vi "禹山叶绿素a校准.vi"() -> ()   [LabVIEW 2016, in "斯坦道多参数.lvlib"]
uses:
  <vilib>/Utility/miscctls.llb/LVPointTypeDef.ctl
  <vilib>/Analysis/NI_AALBase.lvlib
  <vilib>/Analysis/NI_AALPro.lvlib
  <vilib>/Utility/config.llb/NI_LVConfig.lvlib
panel:
  out "第二点校准值":dbl
  out "第一点校准值":dbl
  out "最小值":sgl format="%.2g"
  out "最大值":sgl format="%.2g"
  in  "校准停止":bool
  in  "校准模式":enum16{"两点校准", "单点校准"}(ring)
  in  "标液2":dbl
  in  "标液1":dbl
  out "波形图表":sgl(graph) caption="历史曲线"
  out "温度测量值":dbl caption="温度"
  out "变异系数":dbl format="%.6g"
  out "standard deviation":dbl caption="标准差" format="%0.2f"
  out "mean":dbl caption="均值" format="%0.2f"
  out "提示":string
  in  "校准启动":bool
  out "测试值":dbl
  out "电极斜率":dbl
  out "电极零点":dbl
  # "叶绿素a电极设定"
  # "请选择校准模式:"
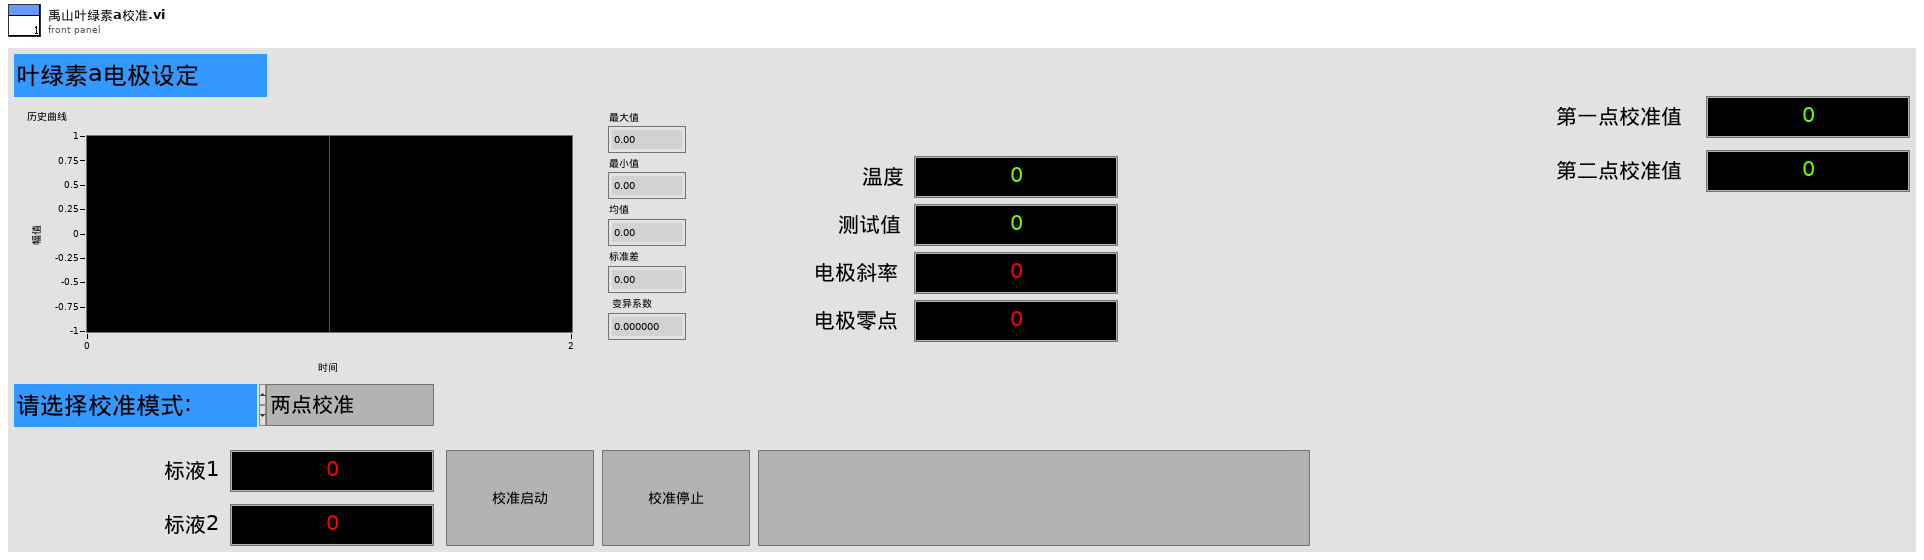
[diagram p1: front panel]
types:
  T1 = typedef "斯坦道多参数.lvlib/校准步骤.ctl" = enum16{"待机", "放置第一点标液", "第一点校准启动", "第一点校准写入", "第一点校准失败", "放置第二点标液", "第二点校准启动", "第二点校准写入", "第二点校准失败", "放置第三点标液", "第三点校准启动", "第三点校准写入", "第三点校准失败", "校准结果写入", "校准结束"}
  T2 = typedef "LVPointTypeDef.ctl" = cluster{"Horizontal":i16, "Vertical":i16}
  T3 = typedef "NI_LVConfig.lvlib/Config Data RefNum.ctl" = refnum<k1>
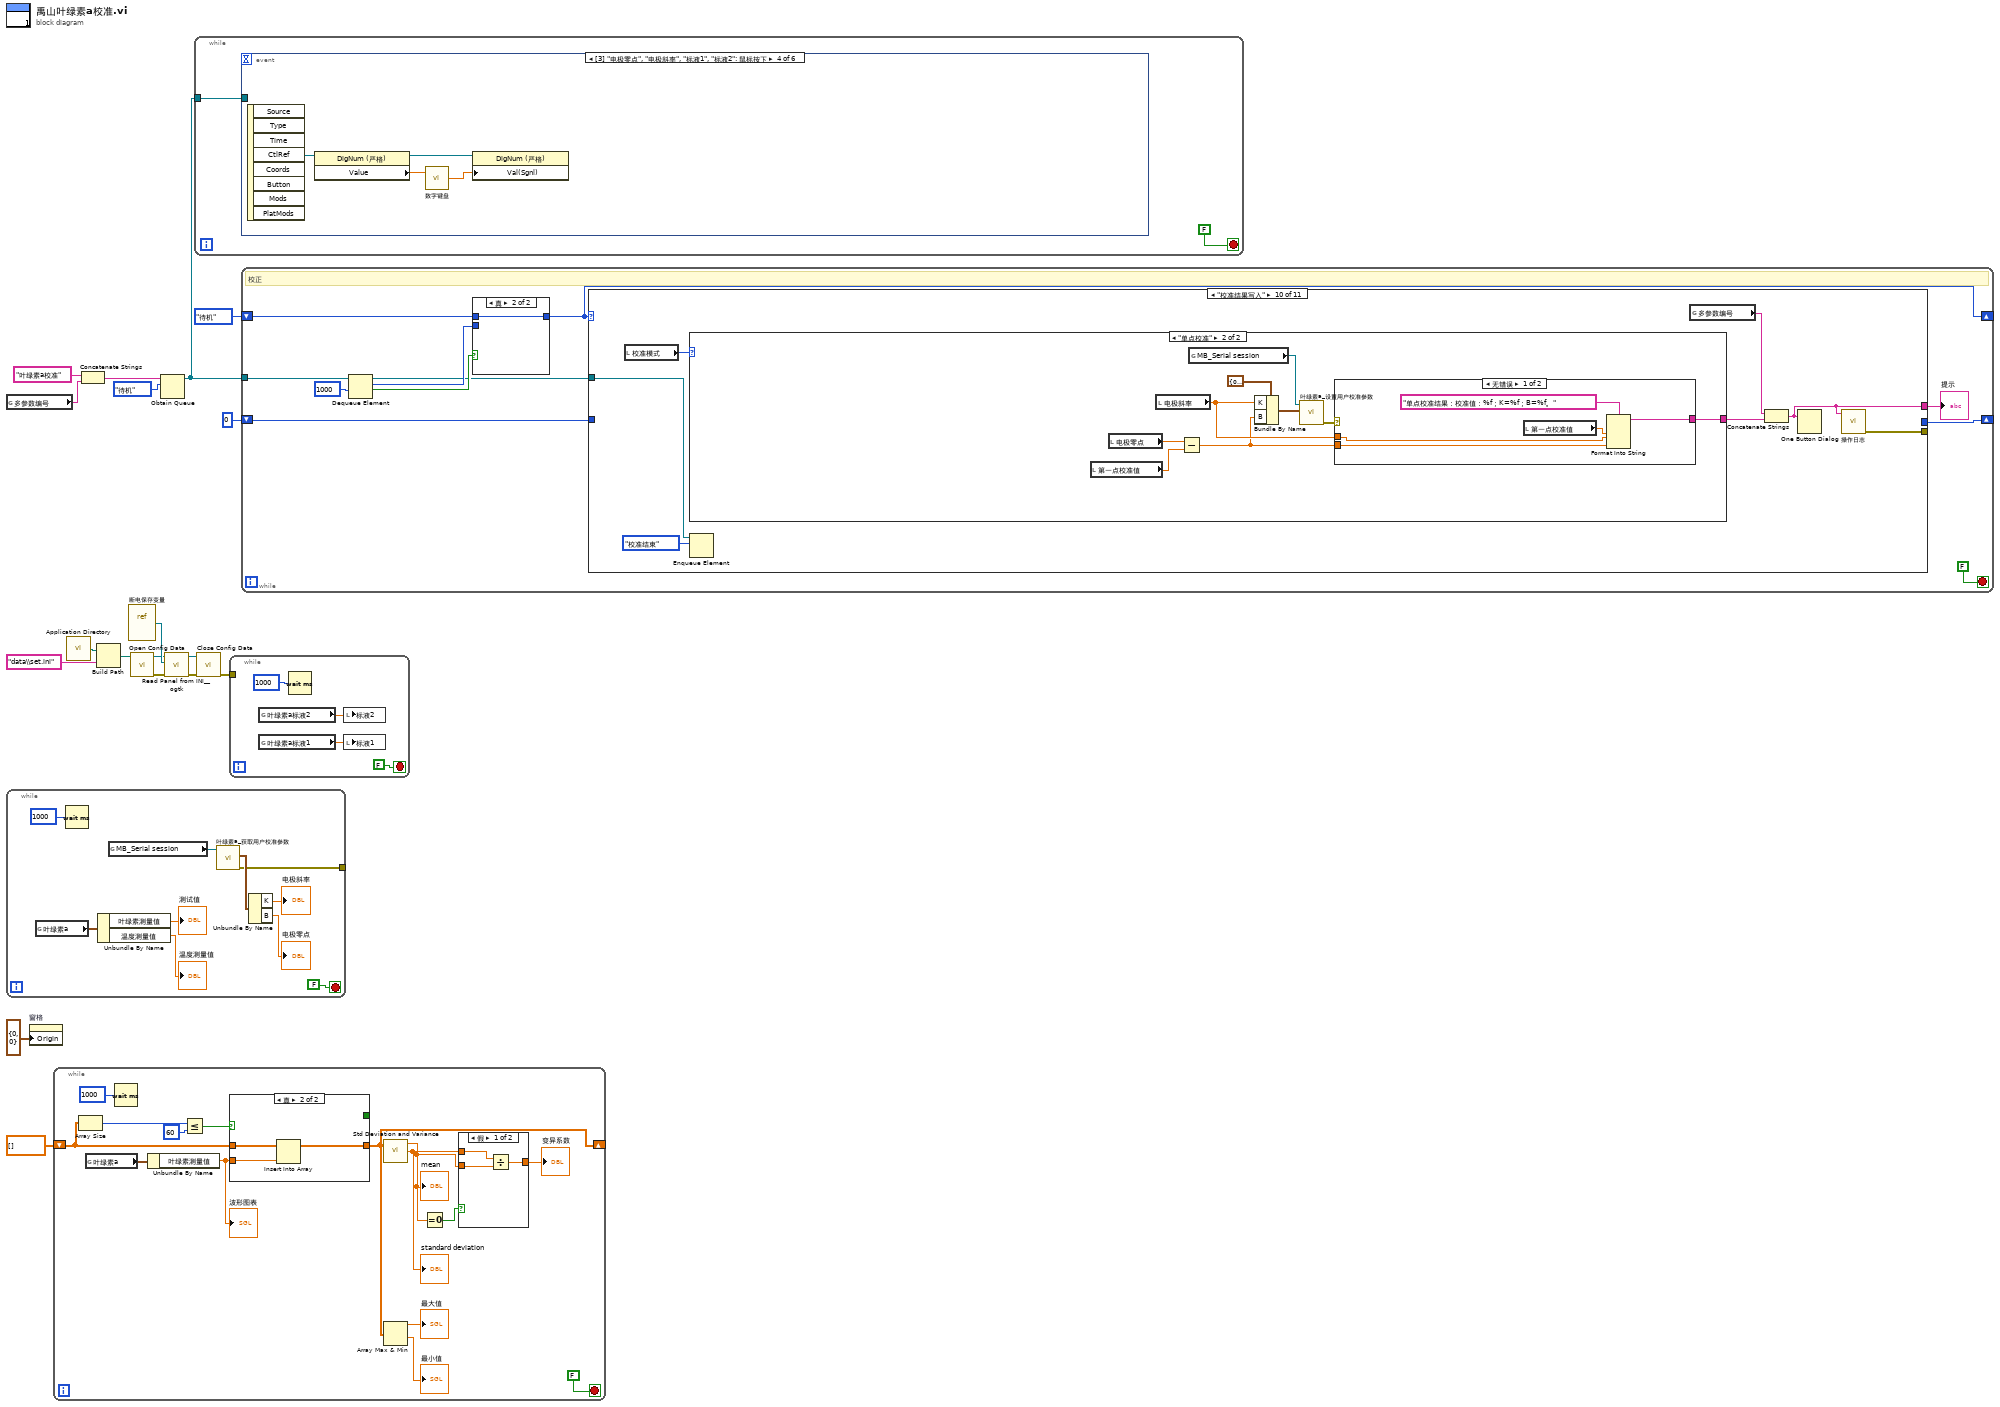
[diagram p0: block diagram]
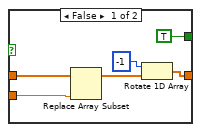
[diagram p3: hidden frame]
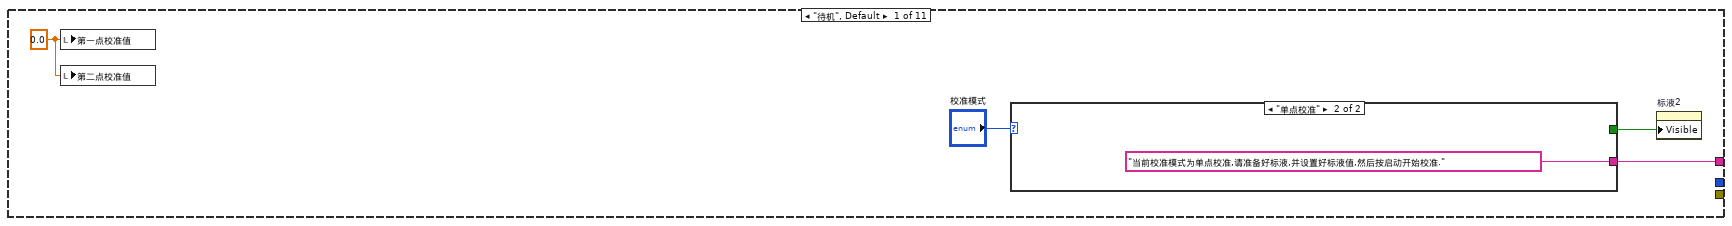
[diagram p5: hidden frame]
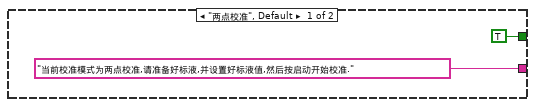
[diagram p6: hidden frame]
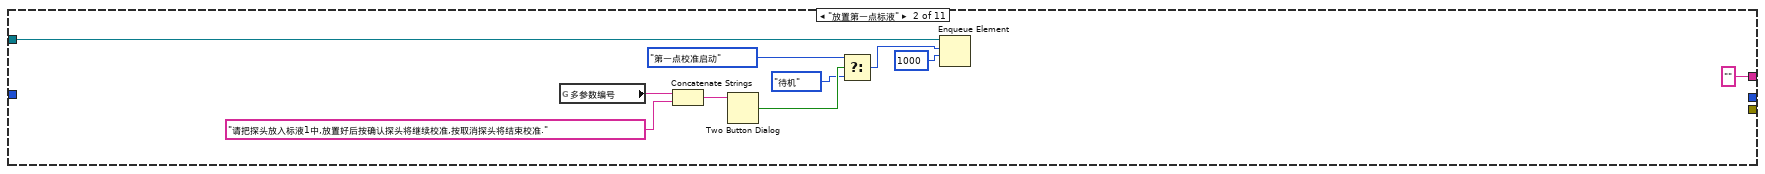
[diagram p7: hidden frame]
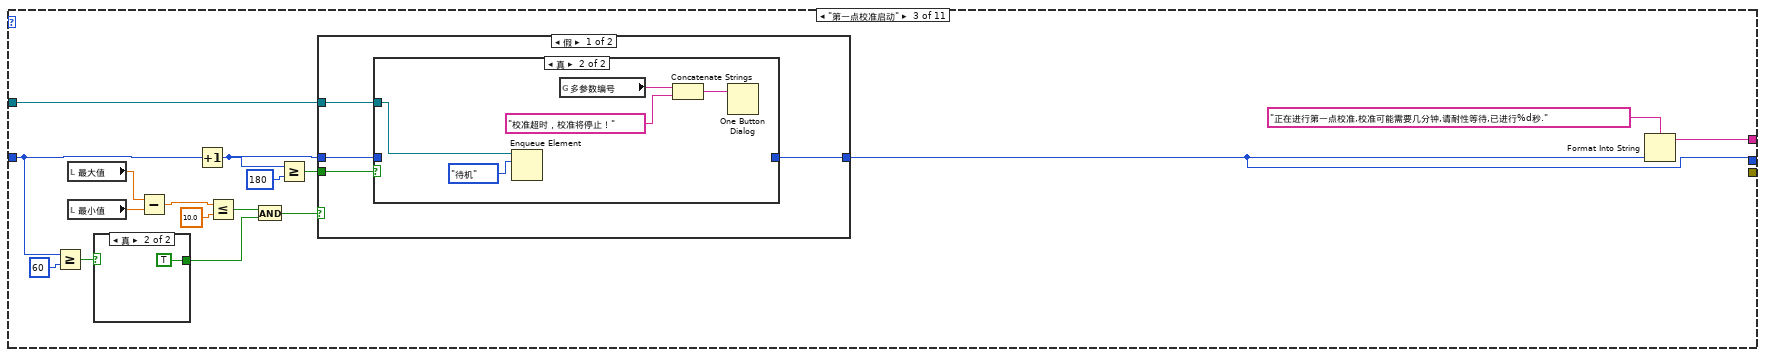
[diagram p8: hidden frame]
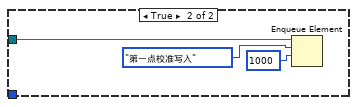
[diagram p10: hidden frame]
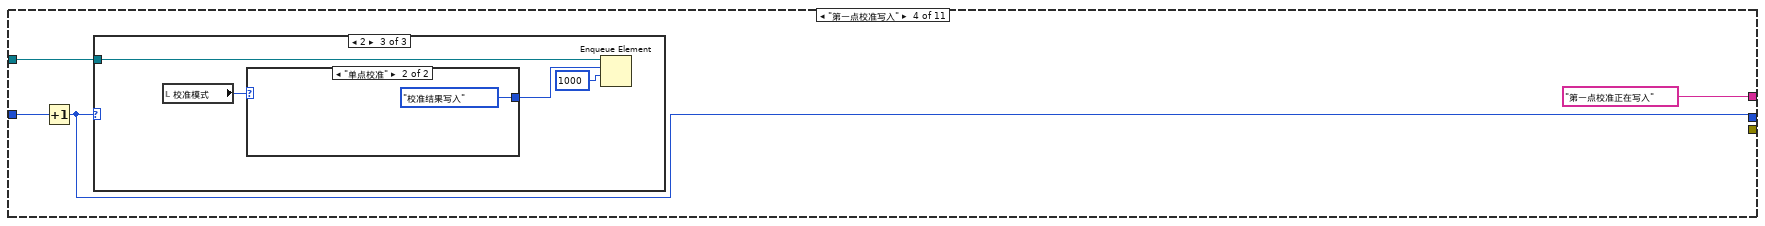
[diagram p12: hidden frame]
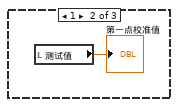
[diagram p14: hidden frame]
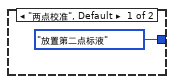
[diagram p15: hidden frame]
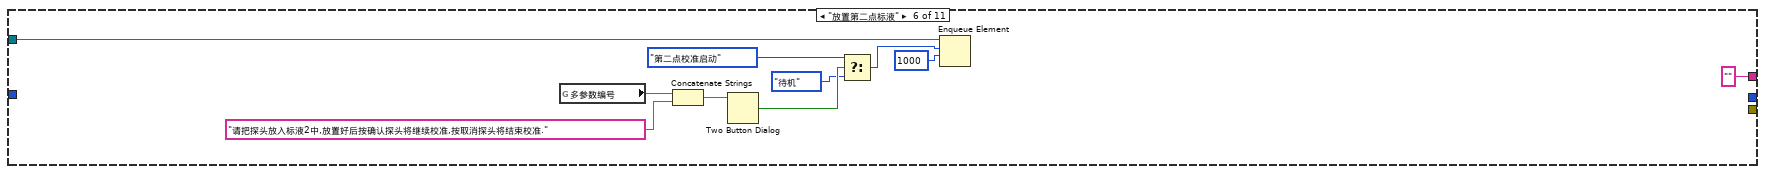
[diagram p17: hidden frame]
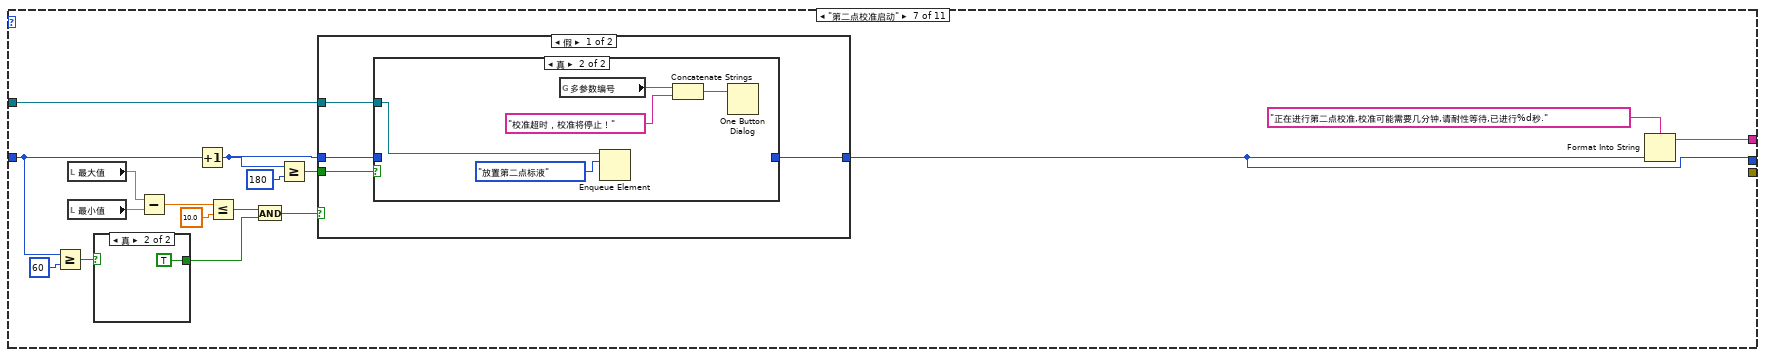
[diagram p18: hidden frame]
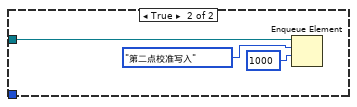
[diagram p20: hidden frame]
diagram:
  n1 = global read "多参数全局变量.vi" "多参数编号"() -> (w1:string)
  n2 = while {
    tunnel: [w23] -> _
    stop <- FALSE stop-if-true
    n3 = global read "禹山过程全局变量.vi" "叶绿素a"() -> (w20:cluster{"温度测量值":sgl, "叶绿素测量值":sgl, "错误标志":u16})
    n4 = Wait (ms)(milliseconds to wait=u32 1000 ("等待时间（毫秒）")) -> ()  [unwired: 1 out]
    n5 = Unbundle By Name(w20) -> ("叶绿素测量值"=→"测试值":sgl, "温度测量值"=→"温度测量值":sgl)
    n6 = global read "多参数全局变量.vi" "MB_Serial session"() -> (w19:refnum<class "MB_Master_Serial.lvclass">)
    n7 = call "叶绿素a_获取用户校准参数.vi"("MB_Serial session in"=w19) -> ("error out"=w23:errorcluster, "输出值"=w26:cluster{"K":sgl, "B":sgl})  [unwired: 8 in, 1 out]
    n8 = Unbundle By Name(w26) -> ("K"=→"电极斜率":sgl, "B"=→"电极零点":sgl)
  }
  n9 = property on="窗格" class="Pane"("Origin"=T2 {"Horizontal"=0, "Vertical"=0} ("原点")) -> ()  [unwired: 2 in, 2 out]
  n10 = while {
    shift-right: [w31] -> _
    shift-left: sgl[] [] -> [w39]
    stop <- FALSE stop-if-true
    n11 = Array Size(array=w39) -> (size(s)=w41:i32)
    n12 = global read "禹山过程全局变量.vi" "叶绿素a"() -> (w33:cluster{"温度测量值":sgl, "叶绿素测量值":sgl, "错误标志":u16})
    n13 = Wait (ms)(milliseconds to wait=u32 1000 ("等待时间（毫秒）")) -> ()  [unwired: 1 out]
    n14 = Unbundle By Name(w33) -> ("叶绿素测量值"=w32:sgl)
    "波形图表" <- w32
    n15 = Less Or Equal?(x=w41, y=60) -> (x <= y?=w40:bool)
    n16 = case shown="真" w40 {
      tunnel: w39 -> [w52 w55]
      tunnel: w32 -> [w50 w54]
      tunnel: [w48 w53] -> w31
      tunnel: [TRUE _] -> _
      frame False {
        n17 = Replace Array Subset(array=w52, new element=w50) -> (w51:sgl[])  [unwired: 1 in]
        n18 = Rotate 1D Array(1:w51, 2:-1 ("n")) -> (0:w48:sgl[])
      }
      frame True {
        n19 = Insert Into Array(array=w55, new element=w54) -> (w53:sgl[])  [unwired: 1 in]
      }
    }
    n20 = call <vilib>:"Std Deviation and Variance.vi"("X"=w31) -> ("mean"=w34:dbl, "standard deviation"=w35:dbl)  [unwired: 1 in, 1 out]
    "standard deviation" <- w35
    "mean" <- w34
    n21 = Array Max & Min(array=w31) -> (max value=→"最大值":sgl, min value=→"最小值":sgl)  [unwired: 2 out]
    n22 = Equal To 0?(x=w34) -> (x = 0?=w38:bool)
    n23 = case shown="假" w38 {
      tunnel: w35 -> [w46 _]
      tunnel: [w45 _] -> w37
      tunnel: w34 -> [w44 _]
      frame False {
        n24 = Divide(x=w46, y=w44) -> (x/y=w45:dbl)
      }
      frame True {
      }
    }
    "变异系数" <- w37
  }
  n25 = call <vilib>:"Application Directory.vi"() -> ("Application Directory"=w8:path)
  n26 = Concatenate Strings("叶绿素a校准" ("名称（未命名）"), w1) -> (w2:string)
  n27 = Build Path(base path=w8, name or relative path="data\\set.ini" ("名称或相对路径")) -> (appended path=w9:path)
  n28 = vi-ref "断电保存变量.vi"() -> (w11:refnum<vi>)
  n29 = call <vilib>:"Open Config Data.vi"("configuration file path"=w9) -> ("error out"=w5:errorcluster, "refnum"=w4:T3)  [unwired: 8 in, 1 out]
  n30 = Obtain Queue(name (unnamed)=w2, element data type=校准步骤."待机" ("枚举")) -> (queue out=w12:refnum<queue>)  [unwired: 3 in, 2 out]
  n31 = call <userlib>:"Read Panel from INI__ogtk.vi"("error in (no error)"=w5, "VI ref"=w11, "refnum"=w4) -> ("error out"=w7:errorcluster, "refnum out"=w6:T3)  [unwired: 7 in]
  n32 = while {
    tunnel: w12 -> [w56]
    stop <- FALSE stop-if-true
    n33 = event shown="[3] \"电极零点\", \"电极斜率\", \"标液1\", \"标液2\": 鼠标按下" {
      selector: _ -> [_ _ _ _ _ _]
      dyn-events: _ -> [_ _ _ _ _ _]
      timeout: _ -> [_ _ _ _ _ _]
      tunnel: w56 -> [_ w59 w63 _ _ _]
      event Timeout {
        n34 = event-data() -> ()  [unwired: 1 in, 3 out]
      }
      event "校准启动": Value Change {
        n35 = event-data() -> ()  [unwired: 1 in, 6 out]
        n36 = Enqueue Element(queue=w59, element=校准步骤."放置第一点标液" ("元素")) -> ()  [unwired: 2 in, 3 out]
      }
      event "校准停止": Value Change {
        n37 = event-data() -> ()  [unwired: 1 in, 6 out]
        n38 = Flush Queue(queue=w63) -> (queue out=w60:refnum<queue>)  [unwired: 1 in, 2 out]
        n39 = Enqueue Element(queue=w60, element=校准步骤."待机" ("元素"), timeout in ms (-1)=1000 ("超时毫秒(-1)")) -> ()  [unwired: 1 in, 3 out]
      }
      event "电极零点", "电极斜率", "标液1", "标液2": Mouse Down {
        n40 = event-data() -> ("CtlRef"=w64:refnum<vi>)  [unwired: 1 in, 7 out]
        n41 = property class="DigNum (严格)"(reference=w64) -> (reference out=w65:refnum<vi>, "Value"=w66:dbl)  [unwired: 1 in, 1 out]
        n42 = call "数字键盘.vi"("OldNumber"=w66) -> ("NewNumber"=w67:dbl)  [unwired: 1 in]
        n43 = property class="DigNum (严格)"(reference=w65, "Val(Sgnl)"=w67) -> ()  [unwired: 1 in, 2 out]
      }
      event "电极零点", "电极斜率": Value Change {
        n44 = event-data() -> ()  [unwired: 1 in, 6 out]
        n45 = local read "电极斜率"() -> (w70:dbl)
        n46 = local read "电极零点"() -> (w69:dbl)
        n47 = global read "多参数全局变量.vi" "MB_Serial session"() -> (w68:refnum<class "MB_Master_Serial.lvclass">)
        n48 = Bundle By Name(cluster=cluster{"K":sgl, "B":sgl} {"K"=0.0, "B"=0.0} ("用户校准参数"), "K"=w70, "B"=w69) -> (w71:cluster{"K":sgl, "B":sgl})
        n49 = call "叶绿素a_设置用户校准参数.vi"("用户校准参数"=w71, "MB_Serial session in"=w68) -> ()  [unwired: 8 in, 2 out]
      }
      event "标液1", "标液2": Value Change {
        n50 = event-data() -> ()  [unwired: 1 in, 6 out]
        n51 = flat-sequence {
          frame #0 {
            n52 = global write "断电保存变量.vi" "叶绿素a标液2"("标液2") -> ()
            n53 = global write "断电保存变量.vi" "叶绿素a标液1"("标液1") -> ()
          }
          frame #1 {
            n54 = call <vilib>:"Application Directory.vi"() -> ("Application Directory"=w84:path)
            n55 = Build Path(base path=w84, name or relative path="data\\set.ini" ("名称或相对路径")) -> (appended path=w83:path)
            n56 = call <vilib>:"Open Config Data.vi"("configuration file path"=w83) -> ("error out"=w87:errorcluster, "refnum"=w88:T3)  [unwired: 8 in, 1 out]
            n57 = vi-ref "断电保存变量.vi"() -> (w81:refnum<vi>)
            n58 = call <userlib>:"Write Panel to INI__ogtk.vi"("error in (no error)"=w87, "VI ref"=w81, "refnum"=w88) -> ("error out"=w85:errorcluster, "refnum out"=w86:T3)  [unwired: 7 in]
            n59 = call <vilib>:"Close Config Data.vi"("error in (no error)"=w85, "refnum"=w86) -> ("error out"=w77:errorcluster, "file path"=w78:path)  [unwired: 8 in]
            n60 = Open/Create/Replace File(file path (use dialog)=w78, error in=w77) -> (refnum out=w79:refnum<file>, error out=w80:errorcluster)  [unwired: 4 in, 1 out]
            n61 = Flush File(refnum=w79, error in=w80) -> (refnum out=w75:refnum<file>, error out=w76:errorcluster)
            n62 = Close File(refnum=w75, error in=w76) -> ()  [unwired: 2 out]
          }
        }
      }
    }
  }
  n63 = call <vilib>:"Close Config Data.vi"("error in (no error)"=w7, "refnum"=w6) -> ("error out"=w3:errorcluster)  [unwired: 8 in, 1 out]
  n64 = while {
    tunnel: w3 -> [_]
    stop <- FALSE stop-if-true
    n65 = global read "断电保存变量.vi" "叶绿素a标液2"() -> (w89:dbl)
    n66 = global read "断电保存变量.vi" "叶绿素a标液1"() -> (w90:dbl)
    n67 = Wait (ms)(milliseconds to wait=u32 1000 ("等待时间（毫秒）")) -> ()  [unwired: 1 out]
    n68 = local write "标液2"(w89) -> ()
    n69 = local write "标液1"(w90) -> ()
  }
  n70 = while "While循环" {
    shift-right: [w94] -> _
    shift-left: 校准步骤."待机" ("枚举") -> [w95]
    shift-right: [w101] -> _
    shift-left: 0 -> [w102]
    tunnel: w12 -> [w99]
    stop <- FALSE stop-if-true
    # "校正"
    n71 = Dequeue Element(queue=w99, timeout in ms (-1)=1000 ("超时毫秒(-1)")) -> (queue out=w93:refnum<queue>, element=w96:T1, timed out?=w97:bool)  [unwired: 1 in, 1 out]
    n72 = case shown="真" w97 {
      tunnel: w96 -> [w104 _]
      tunnel: [w104 w105] -> w94
      tunnel: w95 -> [_ w105]
      frame False {
      }
      frame True {
      }
    }
    n73 = case shown="\"校准结果写入\"" w94 {
      tunnel: [w109 "" ("提示") w138 "第一点校准正在写入" ("提示") _ "" ("提示") w190 "第二点校准正在写入" ("提示") _ w215 w263] -> w100
      tunnel: w102 -> [_ _ w132 w156 _ _ w184 w208 _ _ _]
      tunnel: [_ _ w123 w155 _ _ w175 w207 _ _ _] -> w101
      tunnel: w93 -> [_ w121 w126 w154 _ w173 w178 w206 _ w219 _]
      tunnel: [_ _ _ _ _ _ _ _ _ w214 _] -> _
      frame "待机", Default {
        w106 = 0.0 ("第一点校准值")
        n74 = local write "第一点校准值"(w106) -> ()
        n75 = local write "第二点校准值"(w106) -> ()
        n76 = case shown="\"单点校准\"" "校准模式" {
          tunnel: ["当前校准模式为两点校准,请准备好标液,并设置好标液值,然后按启动开始校准." ("提示") "当前校准模式为单点校准,请准备好标液,并设置好标液值,然后按启动开始校准." ("提示")] -> w109
          tunnel: [TRUE ("可见") _] -> w107
          frame "两点校准", Default {
          }
          frame "单点校准" {
          }
        }
        n77 = property on="标液2" class="DigNum (严格)"("Visible"=w107) -> ()  [unwired: 2 in, 2 out]
      }
      frame "放置第一点标液" {
        n78 = global read "多参数全局变量.vi" "多参数编号"() -> (w113:string)
        n79 = Concatenate Strings(w113, "请把探头放入标液1中,放置好后按确认探头将继续校准,按取消探头将结束校准." ("消息")) -> (w114:string)
        n80 = Two Button Dialog(message=w114) -> (T button?=w119:bool)  [unwired: 2 in]
        n81 = Select(t=校准步骤."第一点校准启动" ("元素"), s=w119, f=校准步骤."待机" ("元素")) -> (s? t:f=w116:T1)
        n82 = Enqueue Element(queue=w121, element=w116, timeout in ms (-1)=1000 ("超时毫秒(-1)")) -> ()  [unwired: 1 in, 3 out]
      }
      frame "第一点校准启动" {
        n83 = Greater Or Equal?(x=w132, y=60) -> (x >= y?=w133:bool)
        n84 = local read "最大值"() -> (w129:sgl)
        n85 = local read "最小值"() -> (w130:sgl)
        n86 = case shown="真" w133 {
          tunnel: [_ TRUE] -> w131
          frame False {
          }
          frame True {
          }
        }
        n87 = Subtract(x=w129, y=w130) -> (x-y=w128:sgl)
        n88 = Increment(x=w132) -> (x+1=w124:i32)
        n89 = Less Or Equal?(x=w128, y=10.0) -> (x <= y?=w136:bool)
        n90 = And(x=w136, y=w131) -> (x .and. y?=w127:bool)
        n91 = Greater Or Equal?(x=w124, y=180) -> (x >= y?=w125:bool)
        n92 = case shown="假" w127 {
          tunnel: w126 -> [w142 w152]
          tunnel: w125 -> [w143 _]
          tunnel: w124 -> [w141 _]
          tunnel: [w140 _] -> w123
          frame False {
            n93 = case shown="真" w143 {
              tunnel: w142 -> [_ w149]
              tunnel: w141 -> [w144 _]
              tunnel: [w144 _] -> w140
              frame False {
              }
              frame True {
                n94 = Enqueue Element(queue=w149, element=校准步骤."待机" ("元素")) -> ()  [unwired: 2 in, 3 out]
                n95 = global read "多参数全局变量.vi" "多参数编号"() -> (w145:string)
                n96 = Concatenate Strings(w145, "校准超时，校准将停止！" ("消息")) -> (w146:string)
                n97 = One Button Dialog(message=w146) -> ()  [unwired: 1 in, 1 out]
              }
            }
          }
          frame True {
            n98 = Enqueue Element(queue=w152, element=校准步骤."第一点校准写入" ("元素"), timeout in ms (-1)=1000 ("超时毫秒(-1)")) -> ()  [unwired: 1 in, 3 out]
          }
        }
        n99 = Format Into String(format string="正在进行第一点校准,校准可能需要几分钟,请耐性等待,已进行%d秒." ("格式字符串"), w123) -> (resulting string=w138:string)  [unwired: 2 in, 1 out]
      }
      frame "第一点校准写入" {
        n100 = Increment(x=w156) -> (x+1=w155:i32)
        n101 = case shown="2" w155 {
          tunnel: w154 -> [_ _ w162]
          frame 0, Default {
          }
          frame 1 {
            n102 = local read "测试值"() -> (→"第一点校准值":dbl)
          }
          frame 2 {
            n103 = local read "校准模式"() -> (w161:enum16{"两点校准", "单点校准"})
            n104 = case shown="\"单点校准\"" w161 {
              tunnel: [校准步骤."放置第二点标液" ("元素") 校准步骤."校准结果写入" ("元素")] -> w160
              frame "两点校准", Default {
              }
              frame "单点校准" {
              }
            }
            n105 = Enqueue Element(queue=w162, element=w160, timeout in ms (-1)=1000 ("超时毫秒(-1)")) -> ()  [unwired: 1 in, 3 out]
          }
        }
      }
      frame "第一点校准失败" {
      }
      frame "放置第二点标液" {
        n106 = global read "多参数全局变量.vi" "多参数编号"() -> (w165:string)
        n107 = Concatenate Strings(w165, "请把探头放入标液2中,放置好后按确认探头将继续校准,按取消探头将结束校准." ("消息")) -> (w166:string)
        n108 = Two Button Dialog(message=w166) -> (T button?=w171:bool)  [unwired: 2 in]
        n109 = Select(t=校准步骤."第二点校准启动" ("元素"), s=w171, f=校准步骤."待机" ("元素")) -> (s? t:f=w168:T1)
        n110 = Enqueue Element(queue=w173, element=w168, timeout in ms (-1)=1000 ("超时毫秒(-1)")) -> ()  [unwired: 1 in, 3 out]
      }
      frame "第二点校准启动" {
        n111 = Greater Or Equal?(x=w184, y=60) -> (x >= y?=w185:bool)
        n112 = local read "最大值"() -> (w181:sgl)
        n113 = local read "最小值"() -> (w182:sgl)
        n114 = case shown="真" w185 {
          tunnel: [_ TRUE] -> w183
          frame False {
          }
          frame True {
          }
        }
        n115 = Subtract(x=w181, y=w182) -> (x-y=w180:sgl)
        n116 = Increment(x=w184) -> (x+1=w176:i32)
        n117 = Less Or Equal?(x=w180, y=10.0) -> (x <= y?=w188:bool)
        n118 = And(x=w188, y=w183) -> (x .and. y?=w179:bool)
        n119 = Greater Or Equal?(x=w176, y=180) -> (x >= y?=w177:bool)
        n120 = case shown="假" w179 {
          tunnel: w178 -> [w194 w204]
          tunnel: w177 -> [w195 _]
          tunnel: w176 -> [w193 _]
          tunnel: [w192 _] -> w175
          frame False {
            n121 = case shown="真" w195 {
              tunnel: w194 -> [_ w201]
              tunnel: w193 -> [w196 _]
              tunnel: [w196 _] -> w192
              frame False {
              }
              frame True {
                n122 = global read "多参数全局变量.vi" "多参数编号"() -> (w197:string)
                n123 = Enqueue Element(queue=w201, element=校准步骤."放置第二点标液" ("元素")) -> ()  [unwired: 2 in, 3 out]
                n124 = Concatenate Strings(w197, "校准超时，校准将停止！" ("消息")) -> (w198:string)
                n125 = One Button Dialog(message=w198) -> ()  [unwired: 1 in, 1 out]
              }
            }
          }
          frame True {
            n126 = Enqueue Element(queue=w204, element=校准步骤."第二点校准写入" ("元素"), timeout in ms (-1)=1000 ("超时毫秒(-1)")) -> ()  [unwired: 1 in, 3 out]
          }
        }
        n127 = Format Into String(format string="正在进行第二点校准,校准可能需要几分钟,请耐性等待,已进行%d秒." ("格式字符串"), w175) -> (resulting string=w190:string)  [unwired: 2 in, 1 out]
      }
      frame "第二点校准写入" {
        n128 = Increment(x=w208) -> (x+1=w207:i32)
        n129 = case shown="2" w207 {
          tunnel: w206 -> [_ _ w213]
          frame 0, Default {
          }
          frame 1 {
            n130 = local read "测试值"() -> (→"第二点校准值":dbl)
          }
          frame 2 {
            n131 = Enqueue Element(queue=w213, element=校准步骤."校准结果写入" ("元素"), timeout in ms (-1)=1000 ("超时毫秒(-1)")) -> ()  [unwired: 1 in, 3 out]
          }
        }
      }
      frame "第二点校准失败" {
      }
      frame "校准结果写入" {
        n132 = local read "校准模式"() -> (w217:enum16{"两点校准", "单点校准"})
        n133 = case shown="\"单点校准\"" w217 {
          tunnel: [w228 w252] -> w220
          frame "两点校准", Default {
            n134 = local read "第一点校准值"() -> (w239:dbl)
            n135 = local read "第二点校准值"() -> (w238:dbl)
            n136 = local read "标液1"() -> (w236:dbl)
            n137 = local read "标液2"() -> (w235:dbl)
            n138 = Insert Into Array(array=dbl[] [] ("Weight"), new element #1=w236, new element #2=w235) -> (w234:dbl[])  [unwired: 1 in]
            n139 = Insert Into Array(array=dbl[] [] ("Weight"), new element #1=w239, new element #2=w238) -> (w233:dbl[])  [unwired: 1 in]
            n140 = local read "电极零点"() -> (w225:dbl)
            n141 = call <vilib>:"Linear Fit.vi"("Y"=w234, "X"=w233) -> ("slope"=w224:dbl, "intercept"=w222:dbl)  [unwired: 9 in, 3 out]
            n142 = local read "电极斜率"() -> (w226:dbl)
            n143 = Multiply(x=w224, y=w225) -> (x*y=w223:dbl)
            n144 = Multiply(x=w226, y=w224) -> (x*y=w227:dbl)
            n145 = Add(x=w222, y=w223) -> (x+y=w221:dbl)
            n146 = global read "多参数全局变量.vi" "MB_Serial session"() -> (w232:refnum<class "MB_Master_Serial.lvclass">)
            n147 = Bundle By Name(cluster=cluster{"K":sgl, "B":sgl} {"K"=0.0, "B"=0.0} ("用户校准参数"), "K"=w227, "B"=w221) -> (w231:cluster{"K":sgl, "B":sgl})
            n148 = call "叶绿素a_设置用户校准参数.vi"("用户校准参数"=w231, "MB_Serial session in"=w232) -> ("error out"=w229:errorcluster)  [unwired: 8 in, 1 out]
            n149 = case shown="无错误" w229 {
              tunnel: w227 -> [w243 _]
              tunnel: w221 -> [w242 _]
              tunnel: [w241 "校准失败"] -> w228
              frame No Error {
                n150 = local read "第一点校准值"() -> (w245:dbl)
                n151 = local read "第二点校准值"() -> (w246:dbl)
                n152 = Format Into String(format string="两点校准结果：第一点校准值：%f；第二点校准值：%f；K=%f；B=%f。" ("提示"), w245, w246, w243, w242) -> (resulting string=w241:string)  [unwired: 2 in, 1 out]
              }
              frame Error {
              }
            }
          }
          frame "单点校准" {
            n153 = local read "第一点校准值"() -> (w250:dbl)
            n154 = local read "电极零点"() -> (w249:dbl)
            n155 = local read "电极斜率"() -> (w251:dbl)
            n156 = Subtract(x=w249, y=w250) -> (x-y=w248:dbl)
            n157 = global read "多参数全局变量.vi" "MB_Serial session"() -> (w256:refnum<class "MB_Master_Serial.lvclass">)
            n158 = Bundle By Name(cluster=cluster{"K":sgl, "B":sgl} {"K"=0.0, "B"=0.0} ("用户校准参数"), "K"=w251, "B"=w248) -> (w255:cluster{"K":sgl, "B":sgl})
            n159 = call "叶绿素a_设置用户校准参数.vi"("用户校准参数"=w255, "MB_Serial session in"=w256) -> ("error out"=w253:errorcluster)  [unwired: 8 in, 1 out]
            n160 = case shown="无错误" w253 {
              tunnel: w251 -> [w259 _]
              tunnel: w248 -> [w258 _]
              tunnel: [w257 "校准失败"] -> w252
              frame No Error {
                n161 = local read "第一点校准值"() -> (w261:dbl)
                n162 = Format Into String(format string="单点校准结果：校准值：%f；K=%f；B=%f。" ("提示"), w261, w259, w258) -> (resulting string=w257:string)  [unwired: 2 in, 1 out]
              }
              frame Error {
              }
            }
          }
        }
        n163 = Enqueue Element(queue=w219, element=校准步骤."校准结束" ("元素")) -> ()  [unwired: 2 in, 3 out]
        n164 = global read "多参数全局变量.vi" "多参数编号"() -> (w216:string)
        n165 = Concatenate Strings(w216, w220) -> (w215:string)
        n166 = One Button Dialog(message=w215) -> ()  [unwired: 1 in, 1 out]
        n167 = call "操作日志.vi"("日志信息"=w215) -> ("error out"=w214:errorcluster)  [unwired: 10 in]
      }
      frame "校准结束" {
        n168 = local read "提示"() -> (w263:string)
      }
    }
    "提示" <- w100
  }
